vi "Read Set Device Parameter Status.vi"(11 "Set Device Parameter Status Msg in":refnum<class "Set Device Parameter Status Msg.lvclass">) -> (0 "error":string, 1 "Status":T1, 2 "Parameter Name":string, 3 "IED Name":string, 5 "Set Device Parameter Status Msg out":refnum<class "Set Device Parameter Status Msg.lvclass">)   [LabVIEW 2015, in "SCADA Core.lvlib" / "Set Device Parameter Status Msg.lvclass"]
uses:
  Set Device Parameter Status Msg.lvclass
  Set Device Parameter Status.ctl
  Set Device Parameter Status Msg.lvclass/Set Device Parameter Status Msg.ctl
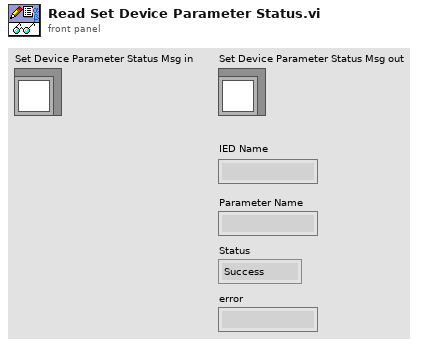
[diagram p1: front panel]
types:
  T1 = typedef "SCADA Core.lvlib/Set Device Parameter Status Msg.lvclass/Set Device Parameter Status.ctl" = enum16{"Success", "Failure"}
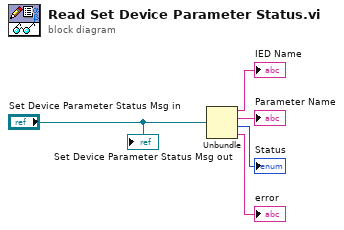
[diagram p0: block diagram]
diagram:
  n1 = Unbundle("Set Device Parameter Status Msg in") -> (→"IED Name":string, →"Parameter Name":string, →"Status":T1, →"error":string)
  "Set Device Parameter Status Msg out" <- "Set Device Parameter Status Msg in"
